vi "LV homework #5 main VI.vi"() -> ()   [LabVIEW 2018]
panel:
  out "LED":bool
  in  "stop":bool
  out "Iteration Count":i32
  out "Results":cluster{"Results #1":dbl[], "Results #2":dbl[]}
  in  "Calculate":bool
  in  "Numeric Inputs":dbl[](array[numeric])
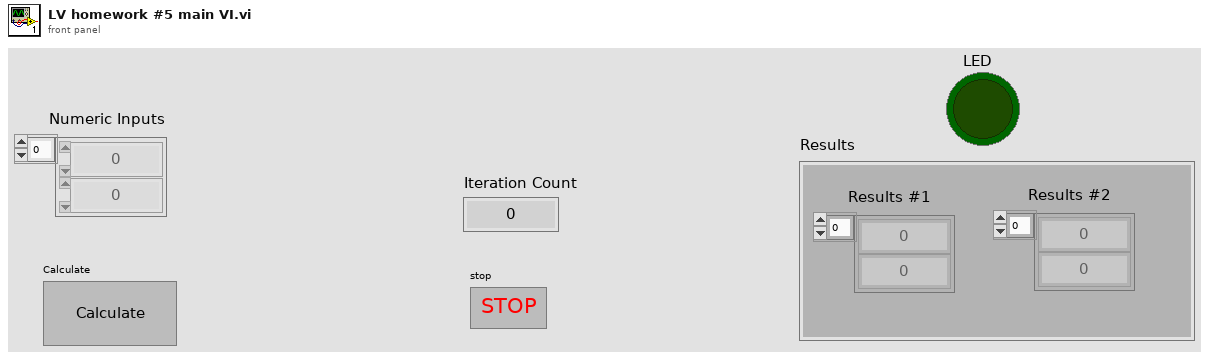
[diagram p1: front panel]
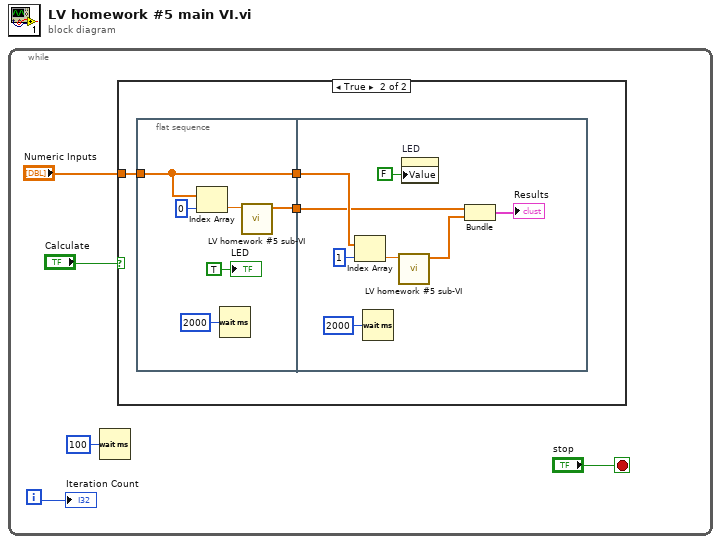
[diagram p0: block diagram]
diagram:
  n1 = while {
    i -> [w1]
    stop <- "stop" stop-if-true
    n2 = Wait (ms)(milliseconds to wait=u32 100) -> ()  [unwired: 1 out]
    n3 = case shown="True" "Calculate" {
      tunnel: "Numeric Inputs" -> [_ w8]
      frame False {
      }
      frame True {
        n4 = flat-sequence {
          tunnel: w8 -> [w12]
          tunnel: [w12] -> w7
          tunnel: [w10] -> w6
          tunnel: w7 -> [w20]
          tunnel: w6 -> [w17]
          frame #0 {
            n5 = Index Array(array=w12, index=0) -> (element=w14:dbl)
            n6 = Wait (ms)(milliseconds to wait=u32 2000) -> ()  [unwired: 1 out]
            n7 = call "LV homework #5 sub-VI.vi"("Numeric Input"=w14) -> ("Results"=w10:dbl[])  [unwired: 10 in]
            "LED" <- TRUE ("LED")
          }
          frame #1 {
            n8 = Index Array(array=w20, index=1) -> (element=w21:dbl)
            n9 = Wait (ms)(milliseconds to wait=u32 2000) -> ()  [unwired: 1 out]
            n10 = call "LV homework #5 sub-VI.vi"("Numeric Input"=w21) -> ("Results"=w16:dbl[])  [unwired: 10 in]
            n11 = property on="LED" class="Bool (strict)"("Value"=FALSE ("LED")) -> ()  [unwired: 2 in, 2 out]
            n12 = Bundle("Results"=w17, "Results"=w16) -> (→"Results":cluster{"Results":dbl[], "Results":dbl[]})  [unwired: 1 in]
          }
        }
      }
    }
    "Iteration Count" <- w1
  }
